vi "QuitDialog.vi"(8 "Error In":errorcluster) -> (0 "Error Out":errorcluster, 3 "OK Clicked?":bool)   [LabVIEW 2017, in "Client.lvlib" / "UI_API.lvlib"]
uses:
  UI_API.lvlib
panel:
  in  "Cancel Button":bool
  in  "OK Button":bool
  # "Are you sure you want to quit?"
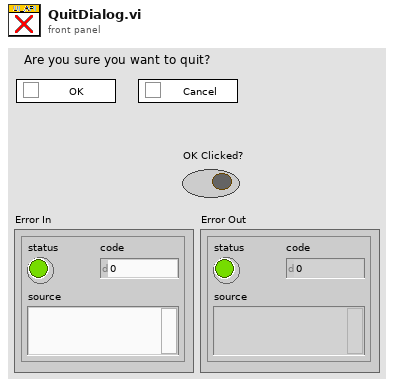
[diagram p1: front panel]
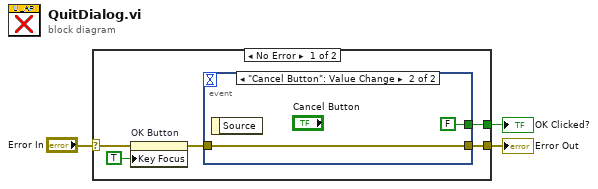
[diagram p0: block diagram]
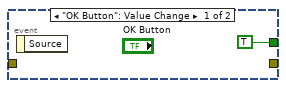
[diagram p2: hidden frame]
diagram:
  n1 = case shown="No Error" "Error In" {
    selector: "Error In" -> [w6 w12]
    tunnel: [w8 _] -> w2
    tunnel: [w4 w12] -> w1
    frame No Error {
      n2 = property on="OK Button" class="Bool"(error in=w6, "Key Focus"=TRUE) -> (error out=w5:errorcluster)  [unwired: 1 in, 1 out]
      n3 = event shown="[1] \"Cancel Button\": Value Change" {
        selector: _ -> [_ _]
        dyn-events: _ -> [_ _]
        timeout: _ -> [_ _]
        tunnel: [TRUE FALSE] -> w8
        tunnel: w5 -> [_ w10]
        tunnel: [_ w10] -> w4
        event "OK Button": Value Change {
          n4 = event-data() -> ()  [unwired: 1 in, 1 out]
        }
        event "Cancel Button": Value Change {
          n5 = event-data() -> ()  [unwired: 1 in, 1 out]
        }
      }
    }
    frame Error {
    }
  }
  "OK Clicked?" <- w2
  "Error Out" <- w1
